vi "Import and Update XML Bookmarks to PDF Report.vi"(0 "PDF path file":path, 7 "PDFCopy":refnum<k24>, 11 "error in (no error)":errorcluster, 13 "Pages [ ] OUT":cluster{"Old":i32, "New":i32}[](array[cluster])) -> (15 "error out":errorcluster)   [LabVIEW 2019, in "Exaprom PDF.lvlib"]
doc: "Version 1.1\nDeveloped by Jean-Marc Simard\nCopyright © 2012, Exaprom Inc.\nAll rights reserved.\nLicense: BSD\n\nWith iTextSharp 4.1.6 (http://itextsharp.sourceforge.net)\nunder Mozilla Public License Version 1.1\n(http://www.mozilla.org/MPL/MPL-1.1.html)"
uses:
  C:/work/niobrara_lv/labview pdf writer fixing/DLL/itextsharp.dll
  DLL/itextsharp.dll
  Controls/File Path Controls/Temporary File.ctl
  Exaprom PDF.lvlib
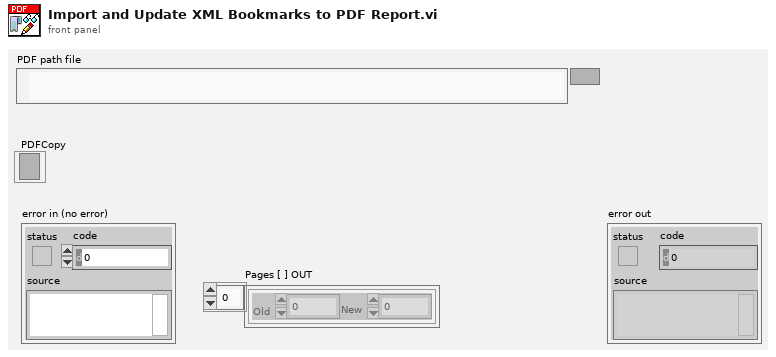
[diagram p1: front panel]
types:
  T1 = typedef "Exaprom PDF.lvlib/Temporary File.ctl" = enum16{".bmp", ".jpeg", ".png", ".pdf", "No File", ".xml"}
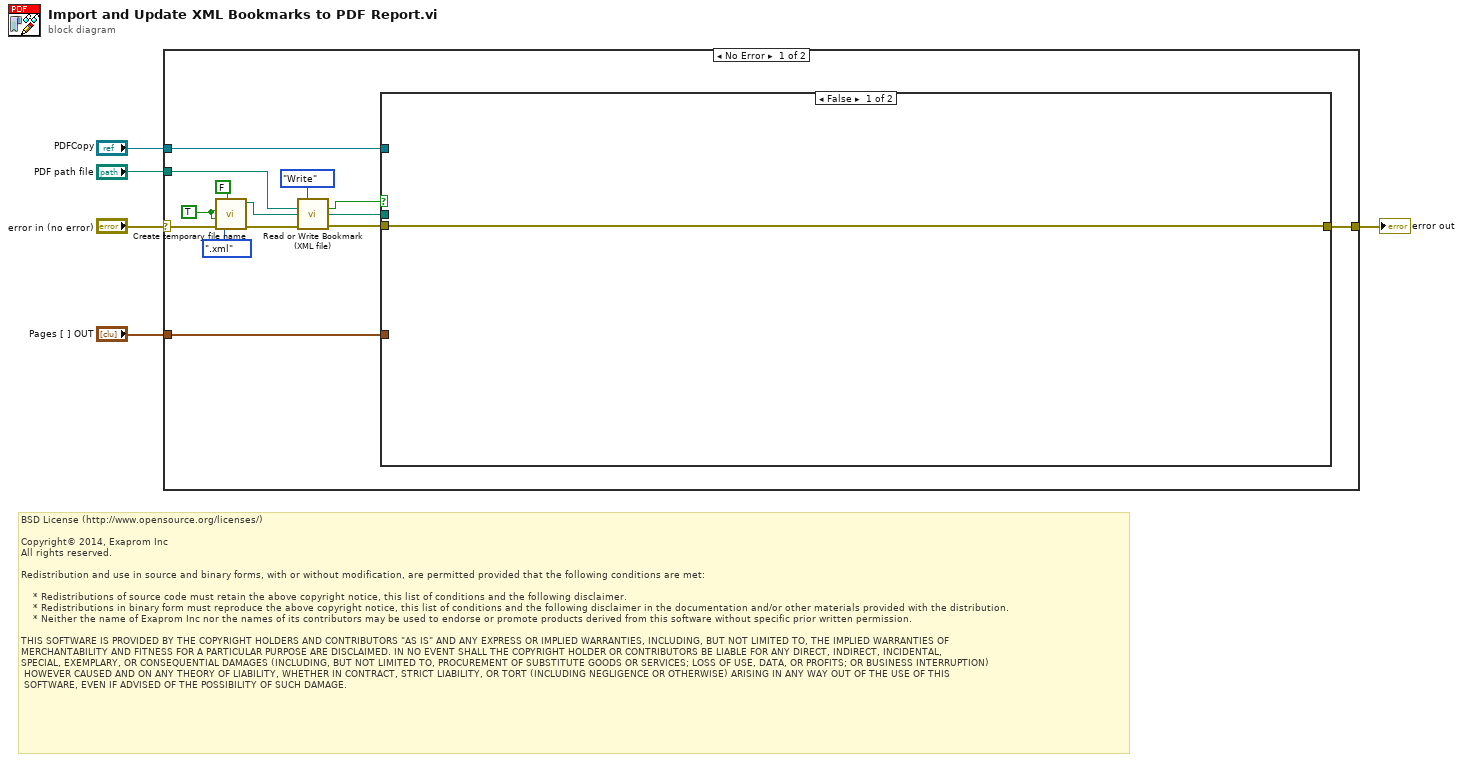
[diagram p0: block diagram]
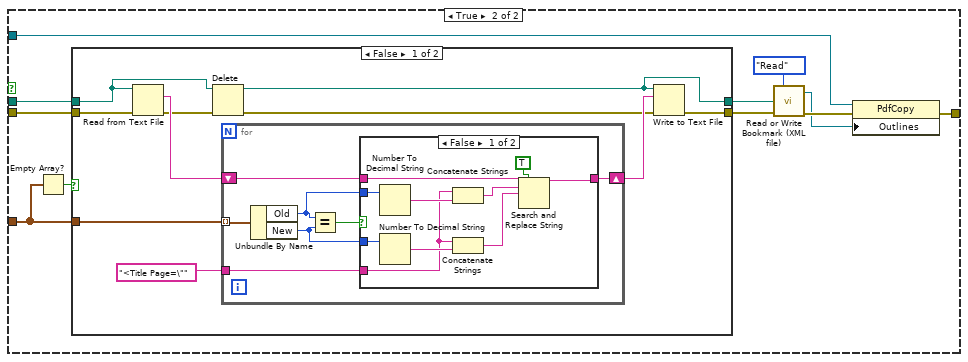
[diagram p2: hidden frame]
diagram:
  # "BSD License (http://www.opensource.org/licenses/)\n\nCopyright© 2014, Exaprom Inc\nAll rights reserved.\n\nRedistribution and use in source and binary forms, with or without modification, are permitted provided that the following conditions are met:\n\n    * Redistributions of source code must retain the above copyright notice, this list of conditions and the following disclaimer.\n    * Redistributions in binary form must reproduce the above copyright notice, this list of conditions and the following disclaimer in the documentation and/or other materials provided with the distribution.\n    * Neither the name of Exaprom Inc nor the names of its contributors may be used to endorse or promote products derived from this software without specific prior written permission.\n\nTHIS SOFTWARE IS PROVIDED BY THE COPYRIGHT HOLDERS AND CONTRIBUTORS \"AS IS\" AND ANY EXPRESS OR IMPLIED WARRANTIES, INCLUDING, BUT NOT LIMITED TO, THE IMPLIED WARRANTIES OF \nMERCHANTABILITY AND FITNESS FOR A PARTICULAR PURPOSE ARE DISCLAIMED. IN NO EVENT SHALL THE COPYRIGHT HOLDER OR CONTRIBUTORS BE LIABLE FOR ANY DIRECT, INDIRECT, INCIDENTAL,\nSPECIAL, EXEMPLARY, OR CONSEQUENTIAL DAMAGES (INCLUDING, BUT NOT LIMITED TO, PROCUREMENT OF SUBSTITUTE GOODS OR SERVICES; LOSS OF USE, DATA, OR PROFITS; OR BUSINESS INTERRUPTION)\n HOWEVER CAUSED AND ON ANY THEORY OF LIABILITY, WHETHER IN CONTRACT, STRICT LIABILITY, OR TORT (INCLUDING NEGLIGENCE OR OTHERWISE) ARISING IN ANY WAY OUT OF THE USE OF THIS\n SOFTWARE, EVEN IF ADVISED OF THE POSSIBILITY OF SUCH DAMAGE."
  n1 = case shown="No Error" "error in (no error)" {
    selector: "error in (no error)" -> [w19 w62]
    tunnel: [w16 w62] -> w5
    tunnel: "PDFCopy" -> [w18 _]
    tunnel: "PDF path file" -> [w17 _]
    tunnel: "Pages [ ] OUT" -> [w7 _]
    frame No Error {
      w14 = TRUE ("hh:mm:ss (false)")
      n2 = call "Create temporary file name.vi"("Temporary Image File"=Temporary_File.".xml", "Flush Files (F)"=FALSE, "error in (no error)"=w19, "msec (F)"=w14, "hh:mm:ss (false)"=w14) -> ("error out"=w10:errorcluster, "File path"=w9:path)  [unwired: 1 in, 4 out]
      n3 = call "Read or Write Bookmark (XML file).vi"("Read or write"=enum16{"Read", "Write"}."Write", "PDF path file"=w17, "XML File"=w9, "error in (no error)"=w10) -> ("Bookmark?"=w6:bool, "XML File duplicate"=w8:path, "error out"=w15:errorcluster)  [unwired: 8 in, 1 out]
      n4 = case shown="False" w6 {
        tunnel: w18 -> [_ w28]
        tunnel: [w20 w27] -> w16
        tunnel: w15 -> [w20 w26]
        tunnel: w8 -> [_ w24]
        tunnel: w7 -> [_ w21]
        frame False {
        }
        frame True {
          n5 = Empty Array?(array=w21) -> (empty?=w22:bool)
          n6 = case shown="False" w22 {
            tunnel: w21 -> [w41 _]
            tunnel: w26 -> [w40 w60]
            tunnel: [w37 w60] -> w25
            tunnel: w24 -> [w34 w61]
            tunnel: [w33 w61] -> w23
            frame False {
              n7 = Read from Text File(file (use dialog)=w34, error in=w40) -> (text=w39:string, error out=w38:errorcluster)  [unwired: 2 in, 2 out]
              n8 = Delete(path (use dialog)=w34, error in=w38) -> (deleted path=w33:path, error out=w35:errorcluster)  [unwired: 3 in, 1 out]
              n9 = for {
                tunnel: w41 -> [w48] mode=indexing
                shift-right: [w46] -> w36
                shift-left: w39 -> [w45]
                tunnel: "<Title Page=\"" -> [w42]
                n10 = Unbundle By Name(w48) -> ("Old"=w44:i32, "New"=w43:i32)
                n11 = Equal?(x=w44, y=w43) -> (x = y?=w47:bool)
                n12 = case shown="False" w47 {
                  tunnel: [w53 w59] -> w46
                  tunnel: w45 -> [w54 w59]
                  tunnel: w44 -> [w58 _]
                  tunnel: w43 -> [w57 _]
                  tunnel: w42 -> [w49 _]
                  frame False {
                    n13 = Number To Decimal String(number=w58) -> (decimal integer string=w56:string)  [unwired: 1 in]
                    n14 = Number To Decimal String(number=w57) -> (decimal integer string=w55:string)  [unwired: 1 in]
                    n15 = Concatenate Strings(w49, w56) -> (w52:string)
                    n16 = Concatenate Strings(w49, w55) -> (w51:string)
                    n17 = Search and Replace String(replace all?=TRUE ("replace all? (F)"), input string=w54, search string=w52, replace string=w51) -> (result string=w53:string)  [unwired: 4 in, 3 out]
                  }
                  frame True {
                  }
                }
              }
              n18 = Write to Text File(file (use dialog)=w33, text=w36, error in=w35) -> (error out=w37:errorcluster)  [unwired: 1 in, 2 out]
            }
            frame True {
            }
          }
          n19 = call "Read or Write Bookmark (XML file).vi"("Read or write"=enum16{"Read", "Write"}."Read", "XML File"=w23, "error in (no error)"=w25) -> ("GetBookmark"=w29:refnum<k24>, "error out"=w30:errorcluster)  [unwired: 9 in, 2 out]
          n20 = property class="PdfCopy"(reference=w28, error in=w30, "Outlines"=w29) -> (error out=w27:errorcluster)  [unwired: 1 out]
        }
      }
    }
    frame Error {
    }
  }
  "error out" <- w5
